vi "LightSheet.vi"() -> ()   [LabVIEW 2015]
uses:
  Camera Properties.ctl
  ModeEnum.ctl
  CameraState.ctl
  Stack_State.ctl
  Stack Track.ctl
  CameraControlTypeDef.ctl
  <vilib>/DAQmx/write.llb/DAQmx Write (Digital 1D Wfm NChan NSamp).vi
  <vilib>/DAQmx/write.llb/DAQmx Write (Analog 1D Wfm NChan NSamp).vi
  <vilib>/DAQmx/create/channels.llb/DAQmx Create Channel (AO-Voltage-Basic).vi
  <vilib>/DAQmx/configure/timing.llb/DAQmx Timing (Sample Clock).vi
  <vilib>/Waveform/DWDTOps.llb/DWDT Uncompress Digital.vi
  <vilib>/DAQmx/miscellaneous.llb/DAQmx Fill In Error Info.vi
  <vilib>/vision/NI_Vision_Development_Module.lvlib
panel:
  in  "Tab Control":enum32{"Camera Settings", "Recording"}(tab)
  in  "Scan":bool
  in  "Scan Continuously":bool
  in  "Camera Mode":T1(ring)
  in  "Slit Width /percent":dbl=100.0
  out "error IO":errorcluster
  in  "V Height":dbl=2048.0 min=4.0 max=2048.0 step=4.0
  in  "V Offset":dbl min=0.0 max=0.0 step=4.0
  in  "H Offset":dbl min=0.0 max=0.0 step=4.0
  in  "H Width":dbl min=4.0 max=2048.0 step=4.0
  in  "Exposure /ms":dbl=40.0 min=0.0010036691729323308 max=10.000004210526315 step=1e-08
  in  "Trigger Source":dbl(ring)=2.0 items=["Internal"=1.0, "External"=2.0]
  in  "Readout Direction":dbl(ring)=2.0 items=["Forward"=1.0, "Backward"=2.0]
  in  "Scanning Mode":dbl(ring)=12.0 items=["Full Frame"=1.0, "Slit Scanning"=12.0]
  in  "Advanced DCAM Controls":i32(listbox) caption="Multicolumn Listbox"
  in  "Mode":T2
  in  "FOV /um":dbl(slide) scale=-10.0..10.0
  in  "Properties":T3=4211904 items=["SENSOR MODE"=4212128, "CCD MODE"=4212384, "READOUT MODE"=4211872, "ACTIVE VIEW INDEX"=4343136, "BITS PER CHANNEL"=4342976, "IMAGE PIXEL TYPE"=4343296, "BINNING"=4215968, "EXPOSURE TIME"=2049184, "CONTRAST GAIN"=3163312, "CONTRAST OFFSET"=3163328, "LIGHT MODE"=2114720, "SENSITIVITY"=2114992, "PHOTON IMAGING MODE"=2115200, "HIGH DYNAMIC RANGE MODE"=3163360, "WHITE BALANCE"=3163568, "TEMPERATURE"=2115232, "TEMPERATURE TARGET"=2115264, "SENSOR COOLER FAN"=2115296, "LINEBUNDLE HEIGHT"=4212192, "MECHANICAL SHUTTER"=2115488, "BACK FOCUS POSITION"=8422304, "TRIGGER CONNECTOR"=1066432, "TRIGGER SOURCE"=1066144, "OUTPUT TRIGGER SOURCE"=1852576, "TRIGGER GLOBAL EXPOSURE"=2049680, "FIRST TRIGGER BEHAVIOR"=2049696, "CHANNEL SYNC"=1852352, "READOUT DIRECTION"=4211904, "PRE HSYNC COUNT"=1852704, "INTERNAL LINE SPEED"=4191408, "INTERNAL LINE INVERVAL"=4191424]
  out "Image":T4(plugin-control)
  out "Histogram":T5(graph)
  in  "stop":bool
  in  "Calibration":bool
  in  "MultiD Scan":bool
  in  "Stage Controller":bool
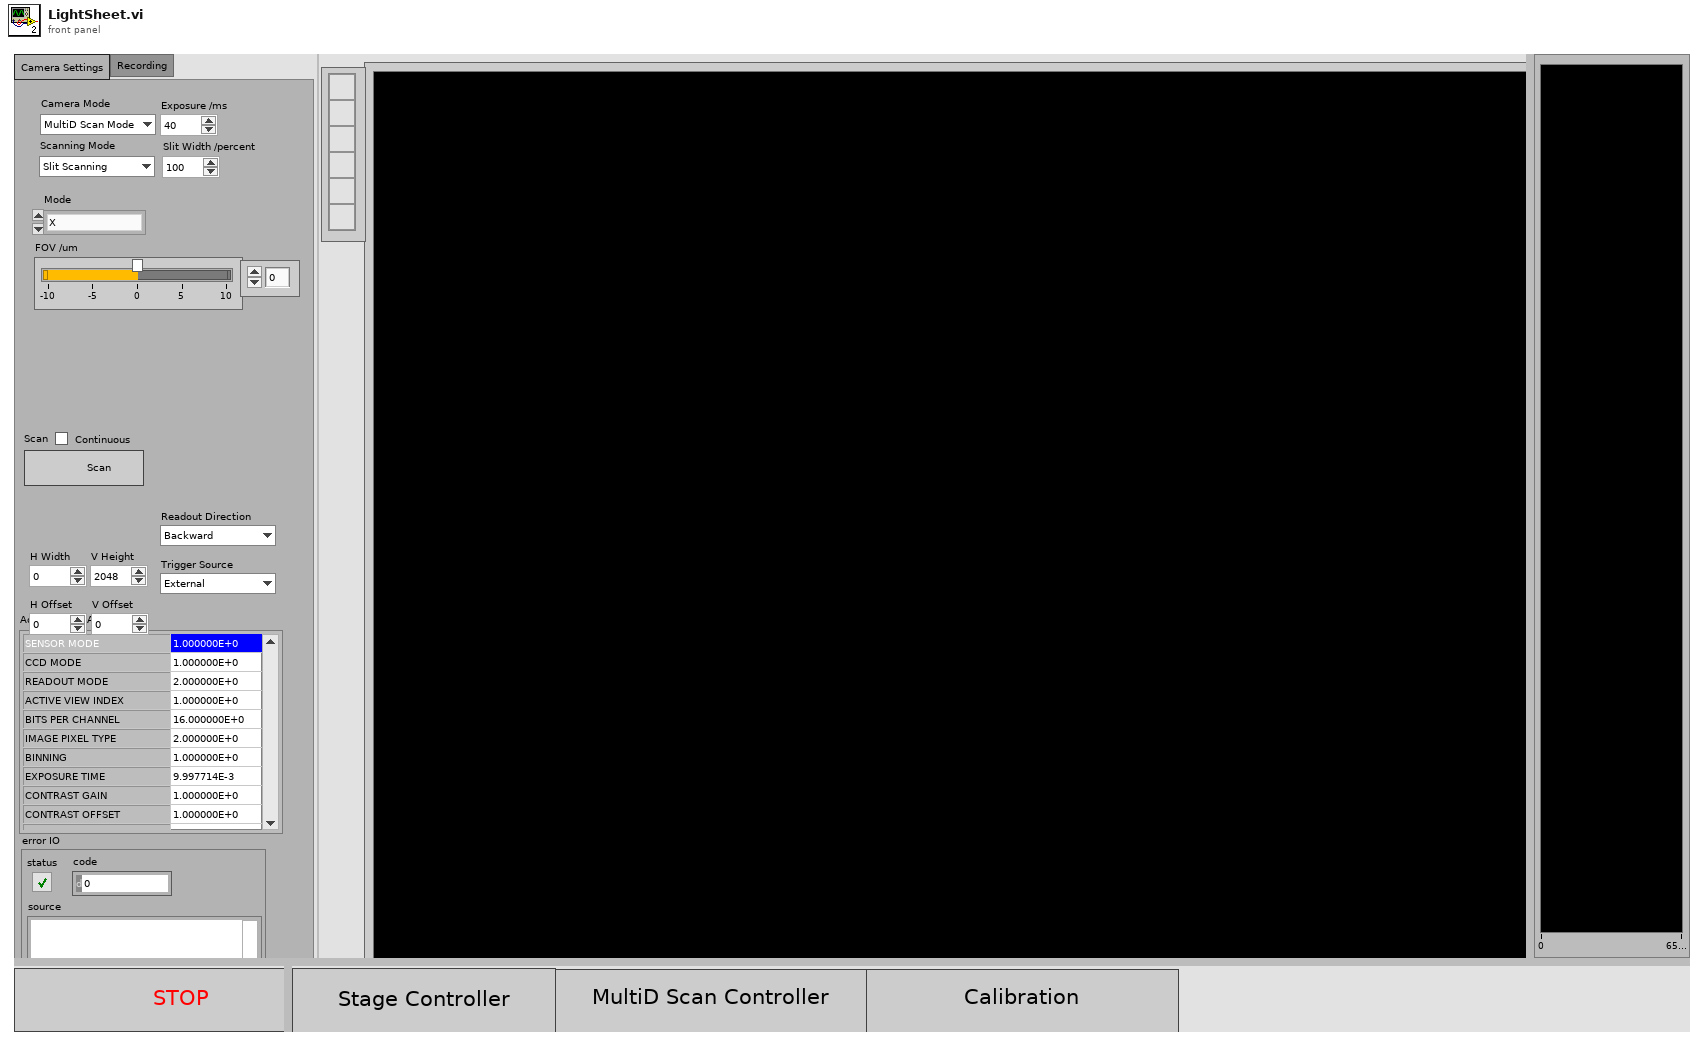
[diagram p1: front panel]
types:
  T1 = enum16{"MultiD Scan Mode", "2D Scan Mode", "Calibration Mode"}
  T2 = typedef "ModeEnum.ctl" = enum16{"X", "XY", "XYZ", "XYZT", "runWaves", "generateWaves", "deInit", "Init", "Idle"}
  T3 = typedef "Camera Properties.ctl" = u32
  T4 = typedef "IMAQ Image.ctl" = refnum<image>
  T5 = cluster{"Starting Value":sgl, "Incremental Value":sgl, "Histogram":u32[]}
  T6 = cluster{"Piezo Position /um":dbl, "Exposure/ms":dbl, "Samples/millisecond":dbl, "Relax/ms":dbl}
  T7 = typedef "CameraControlTypeDef.ctl" = enum16{"IntervalLineInt", "Ram Record", "HardDisk Record", "Disengage Update", "Update", "Idle", "ROI", "Binning", "Scan Mode", "Trigger Mode", "Readout Mode", "Readout Direction", "Preview", "ROIWindow", "Trigger Source"}
  T8 = cluster{"height":u32, "width":u32, "datatype":u32}
  T9 = typedef "Stack_State.ctl" = cluster{"State":T10, "Stack Number":i32, "Image":u16[][], "Stacks":i32}
  T10 = typedef "Stack Track.ctl" = enum16{"Idle", "Display", "Start Sequence", "Read Disk", "STOP", "Collecting", "End"}
  T11 = typedef "CameraState.ctl" = enum16{"init", "active", "deinit"}
  T12 = cluster{"Mode":T2, cluster{"Piezo Position /um":dbl, "Exposure/ms":dbl, "Samples/millisecond":dbl, "Relax/ms":dbl}}
  T13 = typedef "Image Type" = u32
  T14 = cluster{"Value":i32, "Minimum":i32, "Maximum":i32, "Increment":i32}
  T15 = cluster{"Minimum":i32, "Maximum":i32, "Increment":i32}
  T16 = cluster{"Enum":T7, dbl, "timeout in ms (-1)":u32}
  T17 = cluster{"State":T10, "Timeout":i32, "Data 16":u16[][], "Timeout":i32}
  T18 = cluster{"Enum":T7, "Trigger Source":dbl, "timeout in ms (-1)":i32}
  T19 = cluster{"Enum":T7, "Exposure /ms":dbl, "Parameter":u32}
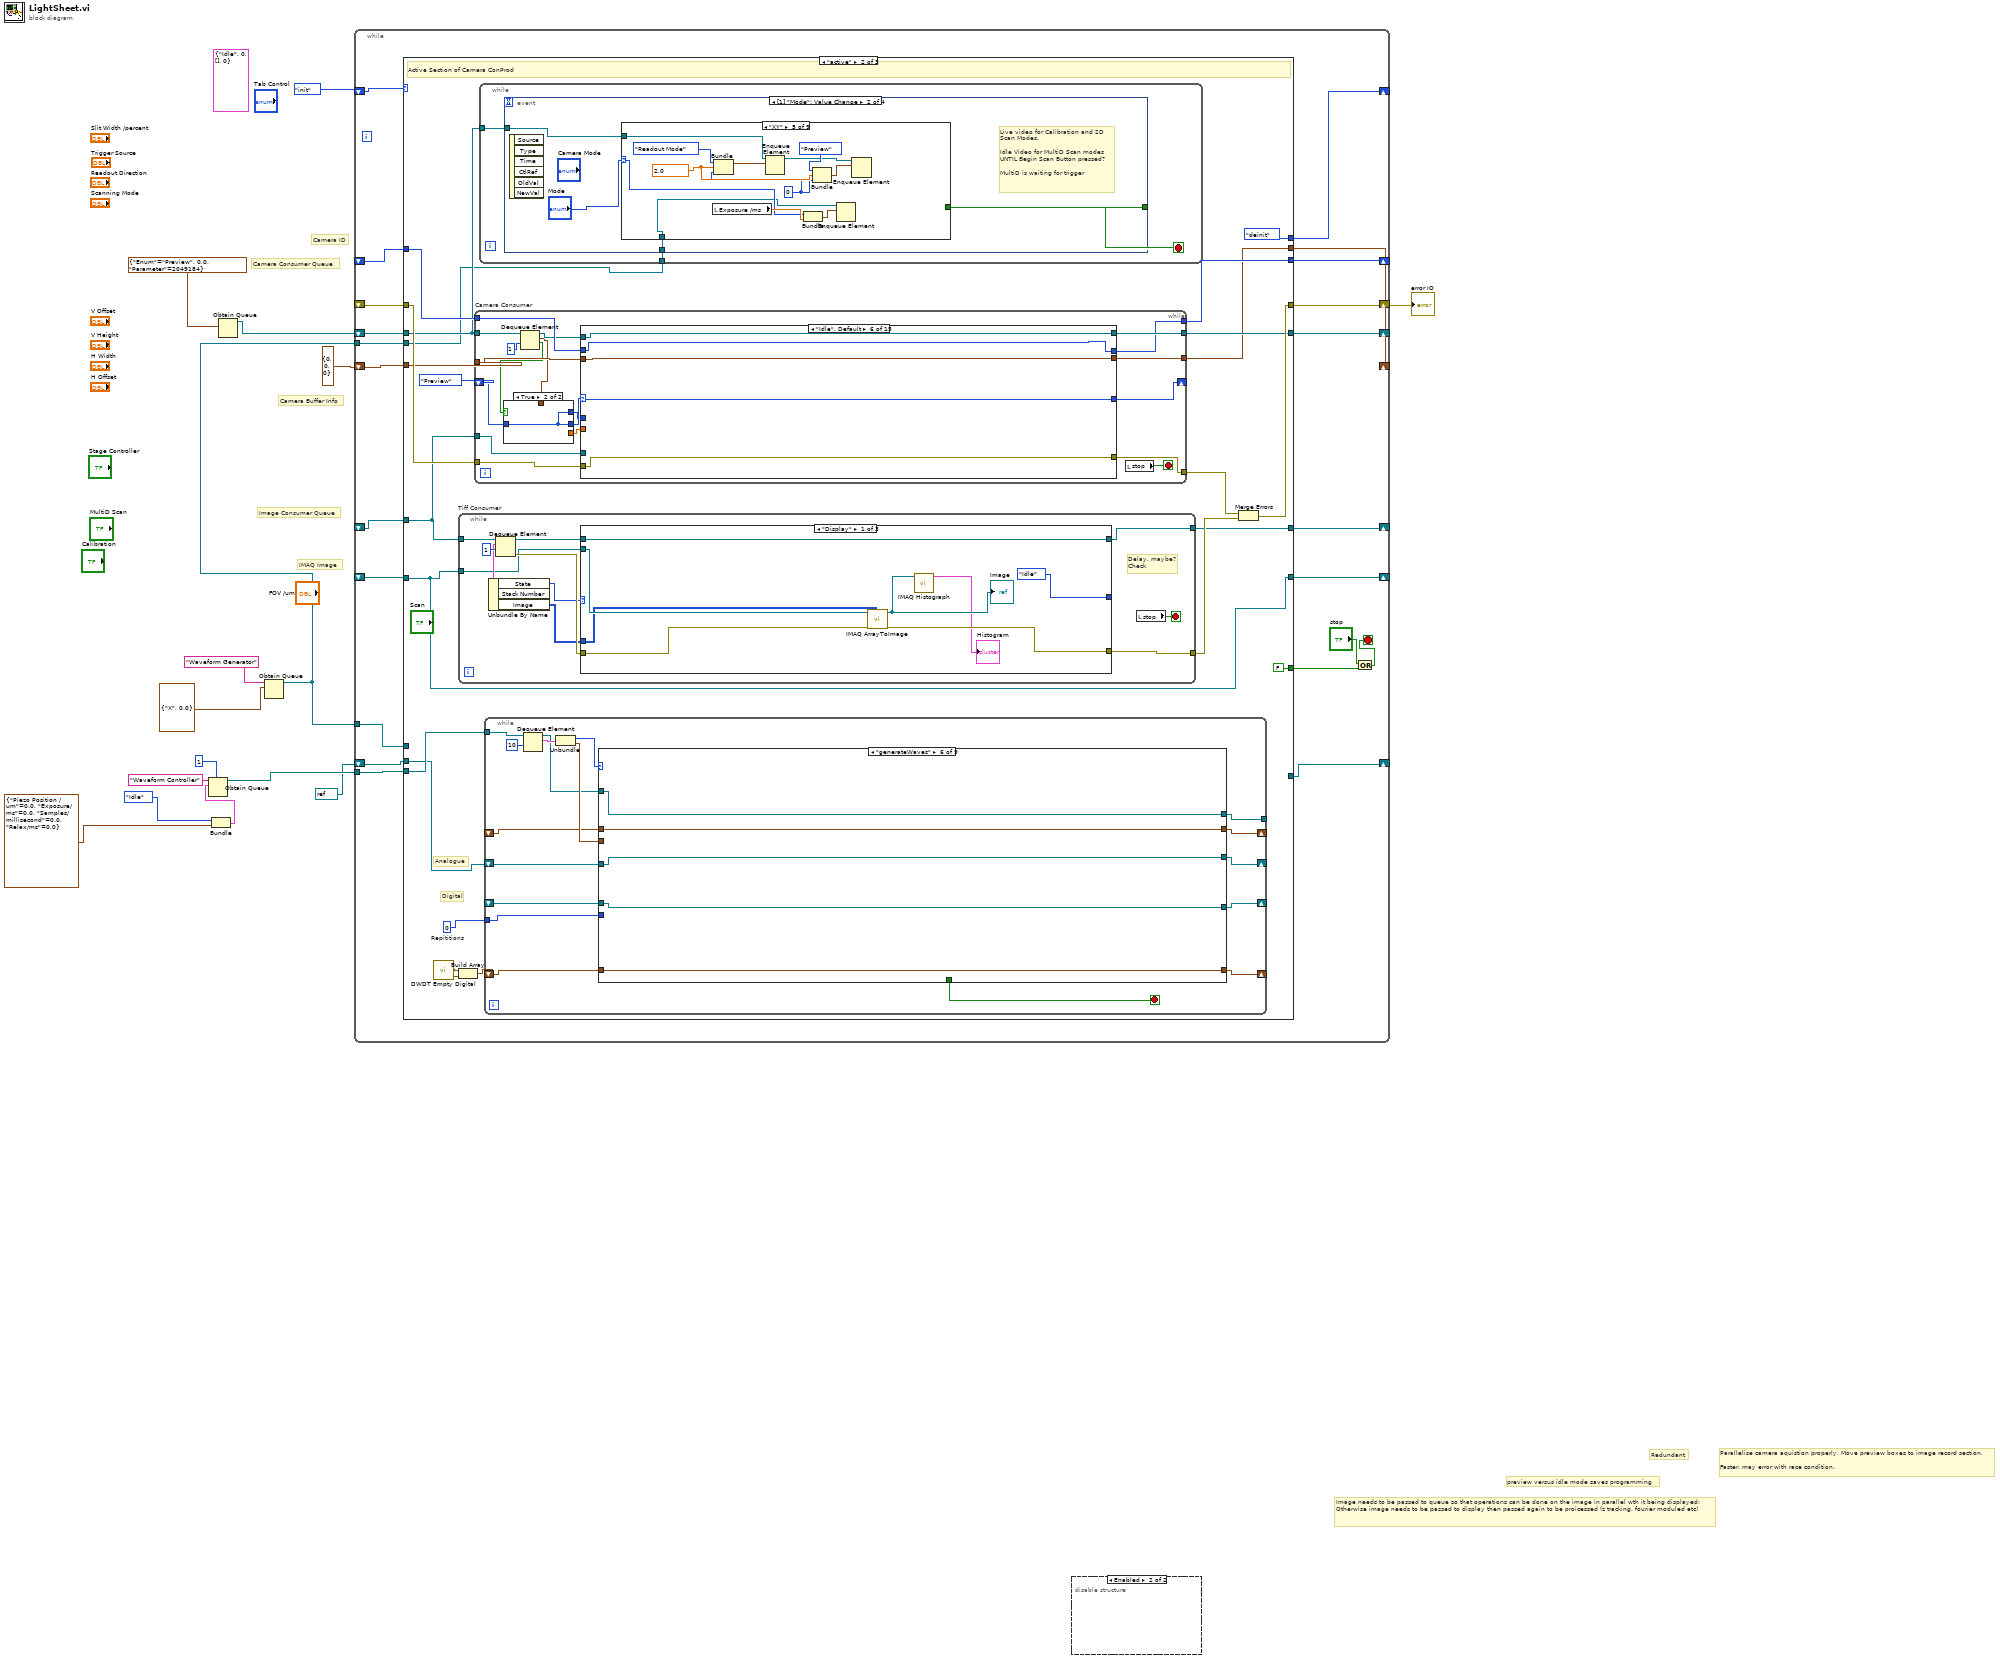
[diagram p0: block diagram]
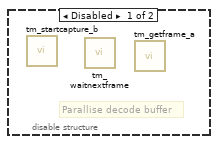
[diagram p2: hidden frame]
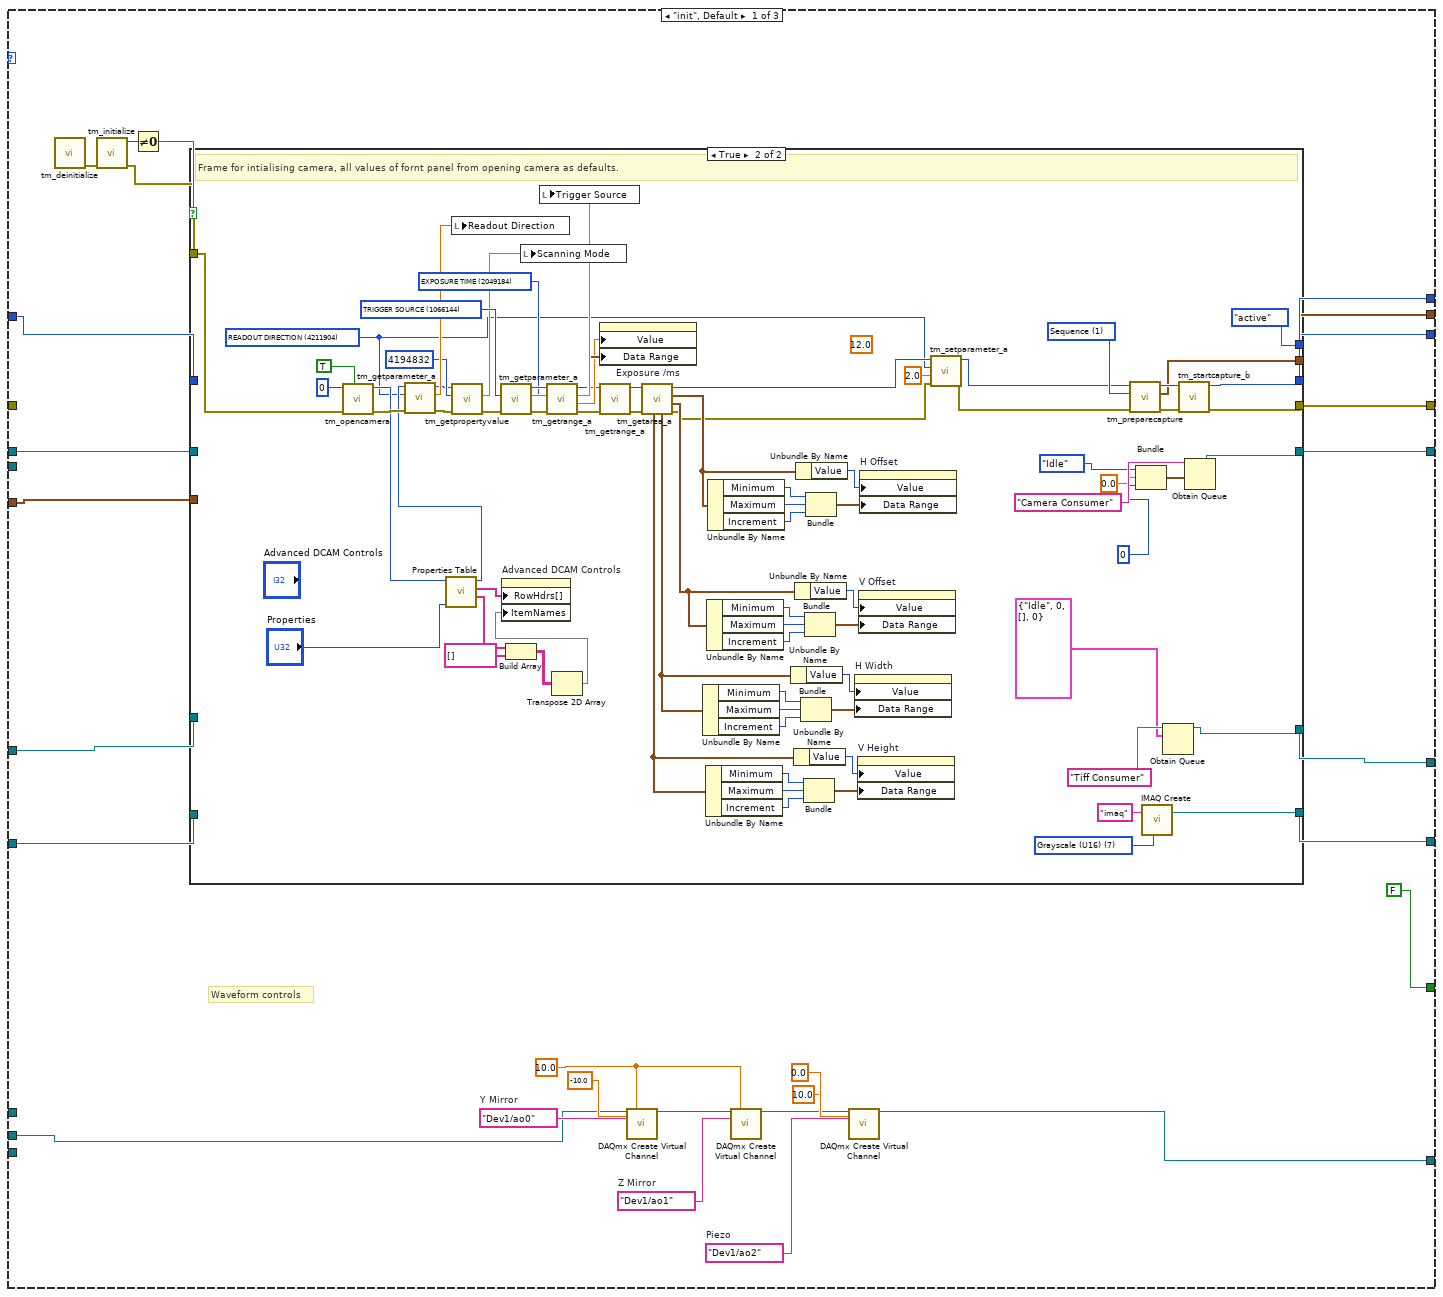
[diagram p3: hidden frame]
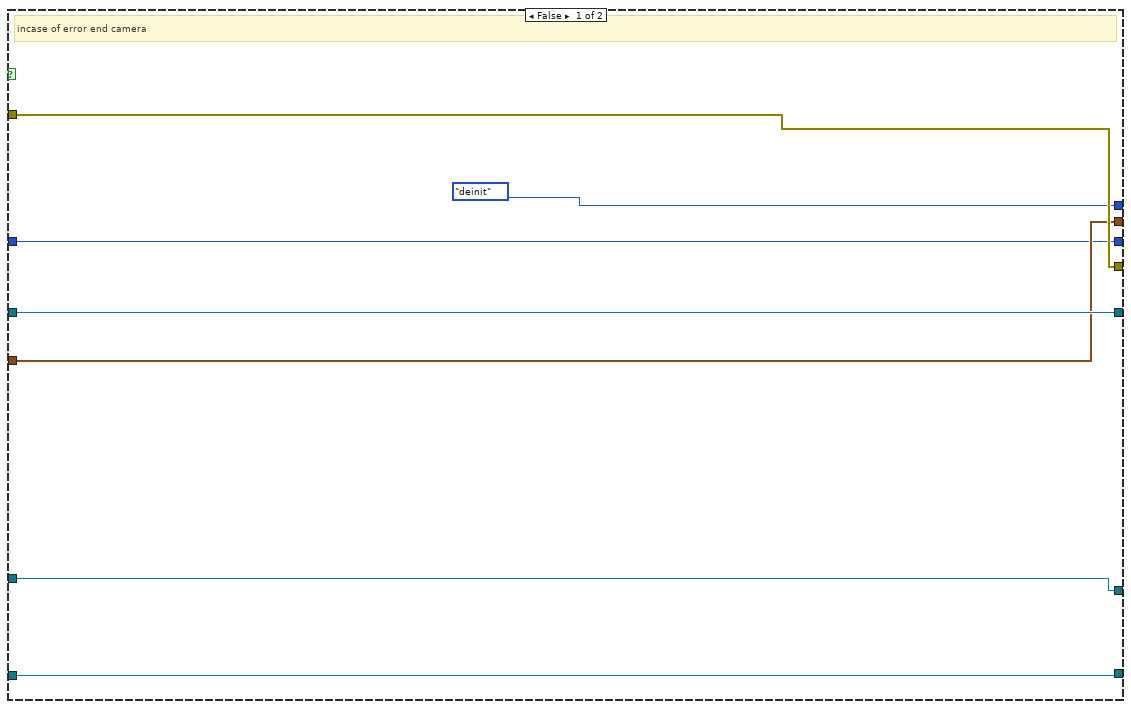
[diagram p4: hidden frame]
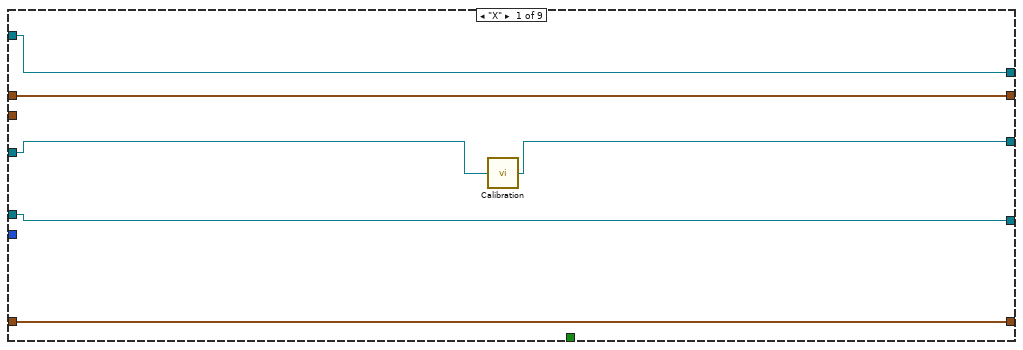
[diagram p5: hidden frame]
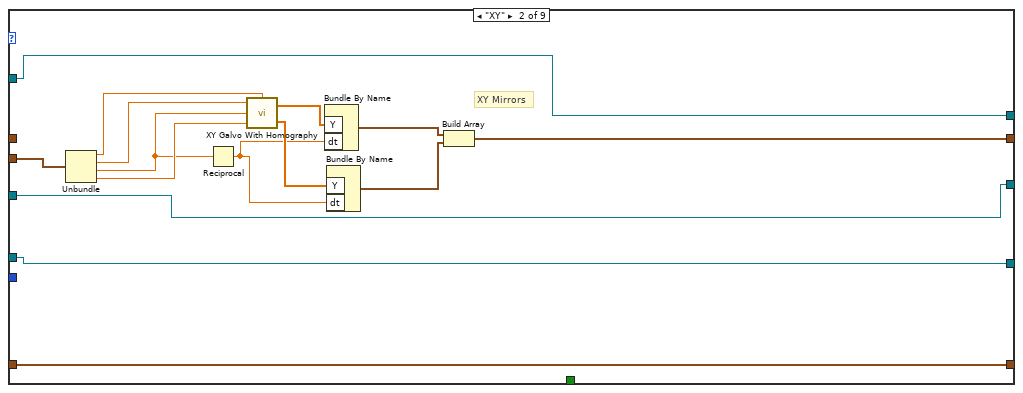
[diagram p6: hidden frame]
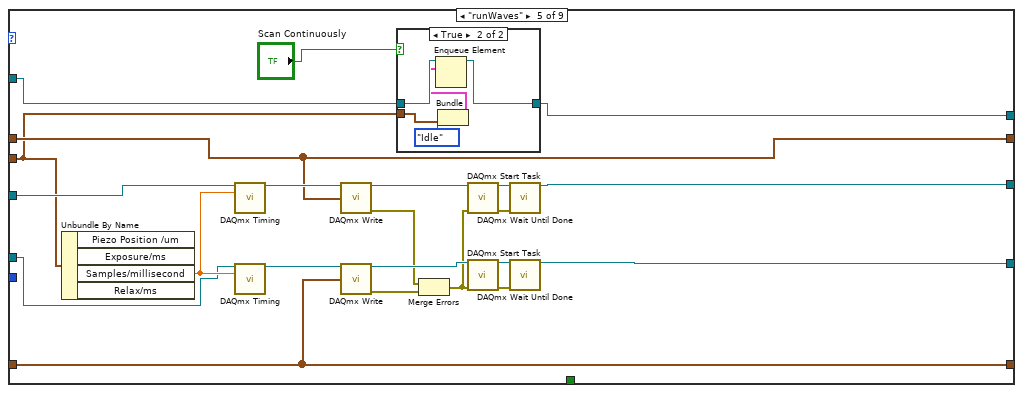
[diagram p9: hidden frame]
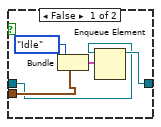
[diagram p10: hidden frame]
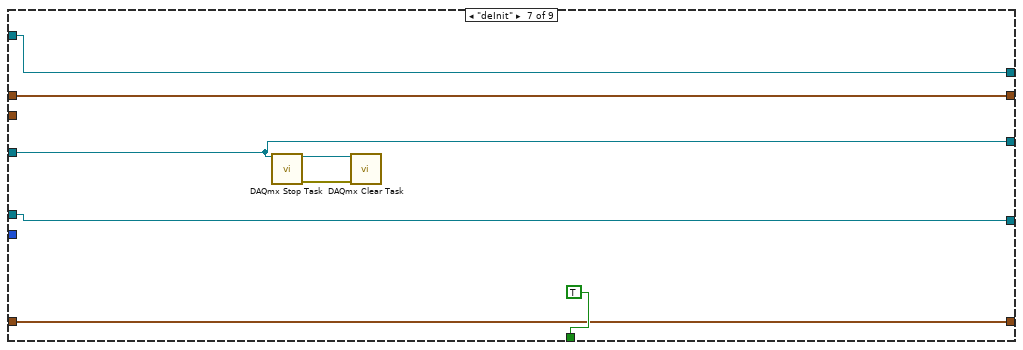
[diagram p11: hidden frame]
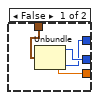
[diagram p16: hidden frame]
diagram:
  (unwired) T9 {"State"=enum."Idle", "Stack Number"=0, "Image"=[], "Stacks"=0} ("input cluster")
  # "IMAQ Image"
  # "Camera Buffer Info"
  # "Image needs to be passed to queue so that operations can be done on the image in parallel wth it being displayed;\nOtherwise image needs to be passed to display then passed again to be proicessed (z tracking, fourier moduled etc)"
  # "preview versus idle mode saves programming"
  # "Parallelise camera aquistion properly. Move preview boxes to image record section.\n\nFaster. may error with race condition."
  # "Redundant"
  # "Image Consumer Queue"
  # "Camera Consumer Queue"
  # "Camera ID"
  n1 = Bundle("Mode"=ModeEnum."Idle", T6 {"Piezo Position /um"=0.0, "Exposure/ms"=0.0, "Samples/millisecond"=0.0, "Relax/ms"=0.0}) -> (w6:T12)  [unwired: 1 in]
  n2 = Obtain Queue(max queue size (-1, unlimited)=1, name (unnamed)="Waveform Controller", element data type=w6) -> (queue out=w3:refnum<queue>)  [unwired: 2 in, 2 out]
  n3 = Obtain Queue(element data type=cluster{"Enum":T7, dbl, "Parameter":u32} {"Enum"=enum."Preview", 0.0, "Parameter"=2049184}) -> (queue out=w10:refnum<queue>)  [unwired: 4 in, 2 out]
  n4 = Obtain Queue(name (unnamed)="Waveform Generator", element data type=cluster{"Mode":T2, "Exposure":dbl} {"Mode"=enum."X", "Exposure"=0.0}) -> (queue out=w9:refnum<queue>)  [unwired: 3 in, 2 out]
  n5 = while {
    shift-right: [w37] -> _
    shift-left: CameraState."init" -> [w36]
    shift-right: [w35] -> _
    shift-left: _ -> [w34]
    shift-right: [w33] -> w14
    shift-left: _ -> [w32]
    shift-right: [w30] -> _
    shift-left: _ -> [w29]
    shift-right: [w31] -> _
    shift-left: w10 -> [w28]
    shift-right: [w24] -> _
    shift-left: T8 {"height"=0, "width"=0, "datatype"=0} ("Buffer Info") -> [w23]
    shift-right: [w22] -> _
    shift-left: _ -> [w21]
    tunnel: w9 -> [w20]
    tunnel: w9 -> [w19]
    tunnel: w3 -> [w18]
    shift-right: [w17] -> _
    shift-left: refnum<k21> refnum ("Mirror Z 2") -> [w16]
    stop <- w26 stop-if-true
    n6 = case shown="\"active\"" w36 {
      tunnel: [w61 CameraState."deinit" CameraState."init"] -> w37
      tunnel: [w60 w171 w475] -> w35
      tunnel: w34 -> [w51 w172 w475]
      tunnel: [w59 w170 w478] -> w33
      tunnel: w32 -> [_ w164 w479]
      tunnel: [w58 w167 w472] -> w31
      tunnel: [w57 w166 w473] -> w30
      tunnel: w29 -> [w55 w159 w473]
      tunnel: w28 -> [w56 w157 w472]
      tunnel: [FALSE ("stop") FALSE ("stop") TRUE ("stop")] -> w25
      tunnel: [w53 w162 w470] -> w24
      tunnel: w23 -> [w52 w161 w470]
      tunnel: w21 -> [w49 w158 w469]
      tunnel: [w50 w158 w469] -> w22
      tunnel: w20 -> [_ _ _]
      tunnel: w19 -> [_ w156 _]
      tunnel: [w41 _ w467] -> w17
      tunnel: w18 -> [_ w152 _]
      tunnel: w16 -> [w38 w151 w467]
      frame "init", Default {
        w44 = tag "Dev1/ao2"  # Piezo
        w45 = tag "Dev1/ao1"  # Z Mirror
        w46 = tag "Dev1/ao0"  # Y Mirror
        w48 = 10.0 ("maximum value")
        # "Waveform controls"
        n7 = call "tm_deinitialize.vi"() -> ("error out"=w65:errorcluster)  [unwired: 11 in]
        n8 = call "tm_initialize.vi"("error in (no error)"=w65) -> ("error out"=w62:errorcluster, "Number Of Cameras"=w64:u32)  [unwired: 7 in, 2 out]
        n9 = Not Equal To 0?(x=w64) -> (x != 0?=w63:bool)
        n10 = case shown="True" w63 {
          tunnel: w62 -> [w72 w144]
          tunnel: [CameraState."deinit" CameraState."active"] -> w61
          tunnel: [w72 w127] -> w59
          tunnel: [w67 w125] -> w60
          tunnel: [w70 w99] -> w58
          tunnel: [w69 w97] -> w57
          tunnel: w56 -> [w70 _]
          tunnel: w55 -> [w69 _]
          tunnel: [w68 w87] -> w53
          tunnel: w52 -> [w68 _]
          tunnel: w51 -> [w67 _]
          tunnel: [w66 w84] -> w50
          tunnel: w49 -> [w66 _]
          frame False {
            # "incase of error end camera"
          }
          frame True {
            (unwired) 12.0 ("Value in")
            w86 = T13 7 items=["Grayscale (U8)", "Grayscale (I16)", "Grayscale (SGL)", "Complex (CSG)", "RGB (U32)", "HSL (U32)", "RGB (U64)", "Grayscale (U16)"] ("Image Type")
            w129 = 1 items=["Snap", "Sequence"] ("Capture mode")
            w141 = u32 2049184 items=["SENSOR MODE"=4212128, "CCD MODE"=4212384, "READOUT MODE"=4211872, "ACTIVE VIEW INDEX"=4343136, "BITS PER CHANNEL"=4342976, "IMAGE PIXEL TYPE"=4343296, "BINNING"=4215968, "EXPOSURE TIME"=2049184, "CONTRAST GAIN"=3163312, "CONTRAST OFFSET"=3163328, "LIGHT MODE"=2114720, "SENSITIVITY"=2114992, "PHOTON IMAGING MODE"=2115200, "HIGH DYNAMIC RANGE MODE"=3163360, "WHITE BALANCE"=3163568, "TEMPERATURE"=2115232, "TEMPERATURE TARGET"=2115264, "SENSOR COOLER FAN"=2115296, "LINEBUNDLE HEIGHT"=4212192, "MECHANICAL SHUTTER"=2115488, "BACK FOCUS POSITION"=8422304, "TRIGGER CONNECTOR"=1066432, "TRIGGER SOURCE"=1066144, "OUTPUT TRIGGER SOURCE"=1852576, "TRIGGER GLOBAL EXPOSURE"=2049680, "FIRST TRIGGER BEHAVIOR"=2049696, "CHANNEL SYNC"=1852352, "READOUT DIRECTION"=4211904, "PRE HSYNC COUNT"=1852704, "INTERNAL LINE SPEED"=4191408, "INTERNAL LINE INVERVAL"=4191424] ("Parameter")
            w79 = T3 4211904 items=["SENSOR MODE"=4212128, "CCD MODE"=4212384, "READOUT MODE"=4211872, "ACTIVE VIEW INDEX"=4343136, "BITS PER CHANNEL"=4342976, "IMAGE PIXEL TYPE"=4343296, "BINNING"=4215968, "EXPOSURE TIME"=2049184, "CONTRAST GAIN"=3163312, "CONTRAST OFFSET"=3163328, "LIGHT MODE"=2114720, "SENSITIVITY"=2114992, "PHOTON IMAGING MODE"=2115200, "HIGH DYNAMIC RANGE MODE"=3163360, "WHITE BALANCE"=3163568, "TEMPERATURE"=2115232, "TEMPERATURE TARGET"=2115264, "SENSOR COOLER FAN"=2115296, "LINEBUNDLE HEIGHT"=4212192, "MECHANICAL SHUTTER"=2115488, "BACK FOCUS POSITION"=8422304, "TRIGGER CONNECTOR"=1066432, "TRIGGER SOURCE"=1066144, "OUTPUT TRIGGER SOURCE"=1852576, "TRIGGER GLOBAL EXPOSURE"=2049680, "FIRST TRIGGER BEHAVIOR"=2049696, "CHANNEL SYNC"=1852352, "READOUT DIRECTION"=4211904, "PRE HSYNC COUNT"=1852704, "INTERNAL LINE SPEED"=4191408, "INTERNAL LINE INVERVAL"=4191424] ("Parameter")
            w147 = u32 1066144 items=["SENSOR MODE"=4212128, "CCD MODE"=4212384, "READOUT MODE"=4211872, "ACTIVE VIEW INDEX"=4343136, "BITS PER CHANNEL"=4342976, "IMAGE PIXEL TYPE"=4343296, "BINNING"=4215968, "EXPOSURE TIME"=2049184, "CONTRAST GAIN"=3163312, "CONTRAST OFFSET"=3163328, "LIGHT MODE"=2114720, "SENSITIVITY"=2114992, "PHOTON IMAGING MODE"=2115200, "HIGH DYNAMIC RANGE MODE"=3163360, "WHITE BALANCE"=3163568, "TEMPERATURE"=2115232, "TEMPERATURE TARGET"=2115264, "SENSOR COOLER FAN"=2115296, "LINEBUNDLE HEIGHT"=4212192, "MECHANICAL SHUTTER"=2115488, "BACK FOCUS POSITION"=8422304, "TRIGGER CONNECTOR"=1066432, "TRIGGER SOURCE"=1066144, "OUTPUT TRIGGER SOURCE"=1852576, "TRIGGER GLOBAL EXPOSURE"=2049680, "FIRST TRIGGER BEHAVIOR"=2049696, "CHANNEL SYNC"=1852352, "READOUT DIRECTION"=4211904, "PRE HSYNC COUNT"=1852704, "INTERNAL LINE SPEED"=4191408, "INTERNAL LINE INVERVAL"=4191424] ("Parameter")
            # "Frame for intialising camera, all values of fornt panel from opening camera as defaults."
            n11 = call "tm_opencamera.vi"("Force Open"=TRUE, "error in (no error)"=w144, "Camera Index"=u32 0) -> ("error out"=w148:errorcluster, "Handle out"=w95:u32)  [unwired: 6 in, 1 out]
            n12 = call "Properties Table.vi"("Properties"="Properties", "Handle In"=w95) -> ("Value Stirngs Out"=w92:string[], "Row Headers"=w93:string[], "Handle Out"=w94:u32)  [unwired: 3 in, 1 out]
            n13 = call "tm_getparameter_a.vi"("error in (no error)"=w148, "Parameter"=w79, "Handle in"=w94) -> ("error out"=w130:errorcluster, "Value out"=w145:dbl, "Handle out"=w133:u32)  [unwired: 6 in]
            n14 = local write "Readout Direction"(w145) -> ()
            n15 = call "tm_getpropertyvalue.vi"("error in (no error)"=w130, "Property ID"=u32 4194832, "Handle in"=w133) -> ("error out"=w131:errorcluster, "Value in"=w132:sgl)  [unwired: 6 in, 1 out]
            n16 = call "tm_getparameter_a.vi"("error in (no error)"=w131, "Parameter"=w147) -> ("error out"=w142:errorcluster, "Value out"=w146:dbl, "Handle out"=w143:u32)  [unwired: 7 in]
            n17 = Build Array(w92, string[] [] ("element")) -> (w90:string[][])
            n18 = local write "Scanning Mode"(w132) -> ()
            n19 = local write "Trigger Source"(w146) -> ()
            n20 = call "tm_getrange_a.vi"("error in (no error)"=w142, "Parameter"=w141, "Handle in"=w143) -> ("error out"=w137:errorcluster, "default"=w139:dbl, "Range"=w140:cluster{"min":dbl, "max":dbl, "step":dbl}, "Handle out"=w138:u32)  [unwired: 2 in, 3 out]
            n21 = Transpose 2D Array(2D array=w90) -> (transposed array=w89:string[][])
            n22 = property on="Advanced DCAM Controls" class="MCListbox (strict)"("RowHdrs[]"=w93, "ItemNames"=w89) -> ()  [unwired: 2 in, 2 out]
            n23 = property on="Exposure /ms" class="DigNum (strict)"("Value"=w139, "Data Range"=w140) -> ()  [unwired: 2 in, 2 out]
            n24 = call "tm_getrange_a.vi"("error in (no error)"=w137, "Handle in"=w138) -> ("error out"=w136:errorcluster, "Handle out"=w135:u32)  [unwired: 3 in, 5 out]
            n25 = call "tm_getarea_a.vi"("error in (no error)"=w136, "Handle in"=w135) -> ("error out"=w81:errorcluster, "V Offset"=w101:T14, "H Offset"=w124:T14, "Handle out"=w83:u32, "H Width"=w102:T14, "V Width"=w103:T14)  [unwired: 4 in]
            n26 = Unbundle By Name(w102) -> ("Minimum"=w113:i32, "Maximum"=w112:i32, "Increment"=w111:i32)
            n27 = Unbundle By Name(w103) -> ("Minimum"=w104:i32, "Maximum"=w105:i32, "Increment"=w106:i32)
            n28 = Unbundle By Name(w101) -> ("Minimum"=w114:i32, "Maximum"=w115:i32, "Increment"=w116:i32)
            n29 = Unbundle By Name(w124) -> ("Minimum"=w123:i32, "Maximum"=w122:i32, "Increment"=w121:i32)
            n30 = Unbundle By Name(w102) -> ("Value"=w109:i32)
            n31 = Unbundle By Name(w103) -> ("Value"=w108:i32)
            n32 = Unbundle By Name(w101) -> ("Value"=w118:i32)
            n33 = Unbundle By Name(w124) -> ("Value"=w119:i32)
            n34 = Bundle("Minimum"=w113, "Maximum"=w112, "Increment"=w111) -> (w110:T15)  [unwired: 1 in]
            n35 = Bundle("Minimum"=w104, "Maximum"=w105, "Increment"=w106) -> (w107:T15)  [unwired: 1 in]
            n36 = Bundle("Minimum"=w114, "Maximum"=w115, "Increment"=w116) -> (w117:T15)  [unwired: 1 in]
            n37 = Bundle("Minimum"=w123, "Maximum"=w122, "Increment"=w121) -> (w120:T15)  [unwired: 1 in]
            n38 = property on="H Width" class="DigNum (strict)"("Value"=w109, "Data Range"=w110) -> ()  [unwired: 2 in, 2 out]
            n39 = property on="V Height" class="DigNum (strict)"("Value"=w108, "Data Range"=w107) -> ()  [unwired: 2 in, 2 out]
            n40 = property on="V Offset" class="DigNum (strict)"("Value"=w118, "Data Range"=w117) -> ()  [unwired: 2 in, 2 out]
            n41 = property on="H Offset" class="DigNum (strict)"("Value"=w119, "Data Range"=w120) -> ()  [unwired: 2 in, 2 out]
            n42 = call "tm_setparameter_a.vi"("error in (no error)"=w81, "Value in"=2.0, "Parameter"=w79, "Handle in"=w83) -> ("error out"=w80:errorcluster, "Handle out"=w82:u32)  [unwired: 6 in]
            n43 = call "tm_preparecapture.vi"("error in (no error)"=w80, "Capture mode"=w129, "Handle in"=w82) -> ("error out"=w128:errorcluster, "Buffer Info"=w87:T8, "Handle out"=w126:u32)  [unwired: 5 in, 1 out]
            n44 = Bundle("Enum"=CameraControlTypeDef."Idle", 0.0, "timeout in ms (-1)"=u32 0) -> (w75:T16)  [unwired: 1 in]
            n45 = call "IMAQ Create"("Image Name"="imaq", "Image Type"=w86) -> ("New Image"=w84:T4)  [unwired: 3 in, 1 out]
            n46 = Obtain Queue(name (unnamed)="Tiff Consumer", element data type=T9 {"State"=enum."Idle", "Stack Number"=0, "Image"=[], "Stacks"=0} ("input cluster")) -> (queue out=w97:refnum<queue>)  [unwired: 3 in, 2 out]
            n47 = call "tm_startcapture_b.vi"("error in (no error)"=w128, "Handle in"=w126) -> ("error out"=w127:errorcluster, "Handle out"=w125:u32)  [unwired: 8 in]
            n48 = Obtain Queue(name (unnamed)="Camera Consumer", element data type=w75) -> (queue out=w99:refnum<queue>)  [unwired: 3 in, 2 out]
          }
        }
        n49 = call-poly <vilib>:"DAQmx Create Virtual Channel.vi"("task in"=w38, "maximum value"=w48, "minimum value"=-10.0, "physical channels"=w46) -> ("task out"=w40:refnum<k21>)  [unwired: 10 in, 1 out]
        n50 = call-poly <vilib>:"DAQmx Create Virtual Channel.vi"("task in"=w40, "maximum value"=w48, "physical channels"=w45) -> ("task out"=w39:refnum<k21>)  [unwired: 11 in, 1 out]
        n51 = call-poly <vilib>:"DAQmx Create Virtual Channel.vi"("task in"=w39, "maximum value"=10.0 ("minimum value"), "minimum value"=0.0 ("maximum value"), "physical channels"=w44) -> ("task out"=w41:refnum<k21>)  [unwired: 10 in, 1 out]
      }
      frame "active" {
        w155 = 0  # Repititions
        # "Digital"
        # "Analogue"
        # "Active Section of Camera ConProd"
        n52 = call <vilib>:"DWDT Empty Digital.vi"() -> ("digital waveform out"=w153:digitalwaveform)  [unwired: 5 in]
        n53 = while "Tiff Consumer" {
          tunnel: [w279] -> w169
          tunnel: [w282] -> w166
          tunnel: w159 -> [w284]
          tunnel: w158 -> [w276]
          stop <- w286 stop-if-true
          # "Delay, maybe?\nCheck"
          n54 = Dequeue Element(queue=w284, timeout in ms (-1)=1) -> (queue out=w281:refnum<queue>, element=w283:T9, error out=w280:errorcluster)  [unwired: 1 in, 1 out]
          n55 = Unbundle By Name(w283) -> ("State"=w277:T10, "Image"=w278:u16[][])  [unwired: 1 out]
          n56 = case shown="\"Display\"" w277 {
            selector: w277 -> [_ w297 w298]
            tunnel: [w294 w296 w299] -> w282
            tunnel: w281 -> [w294 w296 w299]
            tunnel: [Stack_Track."Idle" ("State") w297 w298] -> _
            tunnel: w278 -> [w289 _ _]
            tunnel: w276 -> [w293 _ _]
            tunnel: w280 -> [w292 w295 w300]
            tunnel: [w291 w295 w300] -> w279
            frame "Display" {
              n57 = call "IMAQ ArrayToImage"("Image Pixels (U16)"=w289, "error in (no error)"=w292, "Image"=w293) -> ("error out"=w291:errorcluster, "Image Out"=w288:T4)  [unwired: 7 in]
              "Image" <- w288
              n58 = call "IMAQ Histograph"("Image"=w288) -> ("Histogram Graph"=→"Histogram":T5)  [unwired: 7 in, 3 out]
            }
            frame "Idle", Default {
            }
            frame "Start Sequence" {
            }
          }
          n59 = local read "stop"() -> (w286:bool)
        }
        n60 = Build Array(w153, w153) -> (w154:digitalwaveform[])
        n61 = while "Camera Consumer" {
          tunnel: w164 -> [w317]
          tunnel: w172 -> [w314]
          tunnel: [w313] -> w171
          tunnel: [w316] -> w168
          tunnel: w157 -> [w309]
          tunnel: [w318] -> w167
          shift-right: [w315] -> _
          shift-left: CameraControlTypeDef."Preview" ("Enum") -> [w305]
          tunnel: [w312] -> w162
          tunnel: w161 -> [w311]
          tunnel: w159 -> [w304]
          stop <- w319 stop-if-true
          n62 = Dequeue Element(queue=w309, timeout in ms (-1)=1) -> (queue out=w308:refnum<queue>, element=w303:cluster{"Enum":T7, dbl, "Parameter":u32}, timed out?=w307:bool)  [unwired: 1 in, 1 out]
          n63 = case shown="True" w307 {
            tunnel: [w322 w324] -> w306
            tunnel: w305 -> [_ w324]
            tunnel: w303 -> [w323 _]
            tunnel: [w321 _] -> w302
            tunnel: [w320 w324] -> w301
            frame False {
              n64 = Unbundle(w323) -> ("Enum"=w322:T7, w321:dbl, "Parameter"=w320:u32)
            }
            frame True {
            }
          }
          n65 = case shown="\"Idle\", Default" w306 {
            selector: w306 -> [w328 w333 w338 w343 w351 w356 w361 w366 w371 w376 w381 w386 _ w405 _]
            tunnel: w308 -> [w327 w334 w339 w344 w352 w357 w362 w367 w372 w377 w382 w387 w402 w407 w412]
            tunnel: [w327 w334 w339 w344 w352 w357 w362 w367 w372 w377 w382 w387 w402 w407 w412] -> w318
            tunnel: w317 -> [w329 w332 w337 w342 w350 w355 w360 w365 w370 w375 w380 w385 w392 w404 w410]
            tunnel: [w329 w332 w337 w342 w350 w355 w360 w365 w370 w375 w380 w385 w396 w404 w410] -> w316
            tunnel: [w328 w333 w338 w343 w351 w356 w361 w366 w371 w376 w381 w386 CameraControlTypeDef."Preview" ("Enum") w405 CameraControlTypeDef."Preview" ("Enum")] -> w315
            tunnel: w314 -> [w326 w331 w336 w341 w348 w354 w359 w364 w369 w374 w379 w384 w400 w406 w411]
            tunnel: [w326 w331 w336 w341 w347 w354 w359 w364 w369 w374 w379 w384 w398 w406 w411] -> w313
            tunnel: [w325 w330 w335 w340 w349 w353 w358 w363 w368 w373 w378 w383 w394 w403 w409] -> w312
            tunnel: w311 -> [w325 w330 w335 w340 w349 w353 w358 w363 w368 w373 w378 w383 w394 w403 w409]
            tunnel: w304 -> [_ _ _ _ _ _ _ _ _ _ _ _ w393 _ _]
            tunnel: w302 -> [_ _ _ _ w345 _ _ _ _ _ _ _ _ _ _]
            tunnel: w301 -> [_ _ _ _ w346 _ _ _ _ _ _ _ _ _ _]
            frame "IntervalLineInt" {
            }
            frame "Ram Record" {
            }
            frame "HardDisk Record" {
            }
            frame "Disengage Update" {
            }
            frame "Update" {
              n66 = call "tm_setparameter_a.vi"("Value in"=w345, "Parameter"=w346, "Handle in"=w348) -> ("Handle out"=w347:u32)  [unwired: 7 in, 1 out]
            }
            frame "Idle", Default {
            }
            frame "ROI" {
            }
            frame "Binning" {
            }
            frame "Scan Mode" {
            }
            frame "Trigger Mode" {
            }
            frame "Readout Mode" {
            }
            frame "Readout Direction" {
            }
            frame "Preview" {
              w389 = 0 ("Timeout")
              n67 = call "tm_waitnextframe.vi"("error in (no error)"=w392, "Timeout"=3000, "Handle in"=w400) -> ("error out"=w397:errorcluster, "Handle out"=w399:u32)  [unwired: 5 in, 2 out]
              n68 = call "tm_getframe_a.vi"("error in (no error)"=w397, "Buffer Info"=w394, "Handle in"=w399) -> ("error out"=w396:errorcluster, "Data 16"=w390:u16[][], "Handle out"=w398:u32)  [unwired: 4 in, 2 out]
              n69 = Bundle("State"=Stack_Track."Display", "Timeout"=w389, "Data 16"=w390, "Timeout"=w389) -> (w388:T17)  [unwired: 1 in]
              n70 = Enqueue Element(queue=w393, element=w388, error in (no error)=w392) -> ()  [unwired: 1 in, 3 out]
            }
            frame "ROIWindow" {
            }
            frame "Trigger Source" {
              n71 = call "tm_unpreparecapture.vi"() -> ()  [unwired: 10 in, 2 out]
              n72 = call "tm_setparameter_a.vi"() -> ()  [unwired: 10 in, 2 out]
              n73 = call "tm_preparecapture.vi"() -> ()  [unwired: 8 in, 4 out]
            }
          }
          n74 = local read "stop"() -> (w319:bool)
        }
        n75 = while {
          tunnel: w157 -> [w414]
          tunnel: w156 -> [w413]
          stop <- w415 stop-if-true
          n76 = event shown="[1] \"Mode\": Value Change" {
            selector: _ -> [_ _ _ _]
            dyn-events: _ -> [_ _ _ _]
            timeout: _ -> [_ _ _ _]
            tunnel: [w416 w417 _ _] -> w415
            tunnel: w414 -> [_ w420 _ w465]
            tunnel: w413 -> [_ w418 _ w462]
            event "stop": Value Change {
              n77 = event-data() -> ()  [unwired: 1 in, 6 out]
              n78 = local read "stop"() -> (w416:bool)
            }
            event Value Change {
              # "Live video for Calibration and 2D\nScan Modes.\n\nIdle Video for MultiD Scan modes\nUNTIL Begin Scan Button pressed?\n\nMultiD is waiting for trigger"
              n79 = event-data() -> ()  [unwired: 1 in, 6 out]
              n80 = case shown="\"XY\"" "Mode" {
                selector: "Mode" -> [w423 _ _ _ w446 _ _ _ _]
                tunnel: w420 -> [w431 w439 _ _ w455 _ _ _ _]
                tunnel: w418 -> [w424 _ w442 _ w445 _ _ _ _]
                tunnel: [_ _ _ _ _ TRUE FALSE _ _] -> w417
                frame "X" {
                  w425 = 0 ("timeout in ms (-1)")
                  w426 = 1.0 items=["Internal"=1.0, "External"=2.0] ("Trigger Source")
                  n81 = Bundle("Enum"=CameraControlTypeDef."Readout Mode", "Trigger Source"=w426, "timeout in ms (-1)"=w425) -> (w430:T18)  [unwired: 1 in]
                  n82 = Enqueue Element(queue=w431, element=w430) -> (queue out=w428:refnum<queue>)  [unwired: 2 in, 2 out]
                  n83 = Bundle("Enum"=CameraControlTypeDef."Preview", "Trigger Source"=w426, "timeout in ms (-1)"=w425) -> (w429:T18)  [unwired: 1 in]
                  n84 = Bundle("Mode"=w423, "Exposure /ms"=0.0) -> (w422:cluster{"Mode":T2, "Exposure /ms":dbl})  [unwired: 1 in]
                  n85 = Enqueue Element(queue=w428, element=w429) -> ()  [unwired: 2 in, 3 out]
                  n86 = Enqueue Element(queue=w424, element=w422) -> ()  [unwired: 2 in, 3 out]
                }
                frame "XYZ" {
                  w433 = 0 ("timeout in ms (-1)")
                  w434 = 2.0 items=["Internal"=1.0, "External"=2.0] ("Trigger Source")
                  n87 = Bundle("Enum"=CameraControlTypeDef."Readout Mode", "Trigger Source"=w434, "timeout in ms (-1)"=w433) -> (w438:T18)  [unwired: 1 in]
                  n88 = Enqueue Element(queue=w439, element=w438) -> (queue out=w437:refnum<queue>)  [unwired: 2 in, 2 out]
                  n89 = Bundle("Enum"=CameraControlTypeDef."Idle", "Trigger Source"=w434, "timeout in ms (-1)"=w433) -> (w436:T18)  [unwired: 1 in]
                  n90 = Enqueue Element(queue=w437, element=w436) -> ()  [unwired: 2 in, 3 out]
                }
                frame "generateWaves" {
                  w444 = ModeEnum."generateWaves"  # Mode
                  n91 = local read "Exposure /ms"() -> (w443:dbl)
                  n92 = Bundle("Mode"=w444, "Exposure /ms"=w443) -> (w441:cluster{"Mode":T2, "Exposure /ms":dbl})  [unwired: 1 in]
                  n93 = Enqueue Element(queue=w442, element=w441) -> ()  [unwired: 2 in, 3 out]
                }
                frame "XYZT" {
                }
                frame "XY" {
                  w449 = 0 ("timeout in ms (-1)")
                  w450 = 2.0 items=["Internal"=1.0, "External"=2.0] ("Trigger Source")
                  n94 = local read "Exposure /ms"() -> (w447:dbl)
                  n95 = Bundle("Enum"=CameraControlTypeDef."Readout Mode", "Trigger Source"=w450, "timeout in ms (-1)"=w449) -> (w454:T18)  [unwired: 1 in]
                  n96 = Enqueue Element(queue=w455, element=w454) -> (queue out=w451:refnum<queue>)  [unwired: 2 in, 2 out]
                  n97 = Bundle("Mode"=w446, "Exposure /ms"=w447) -> (w448:cluster{"Mode":T2, "Exposure /ms":dbl})  [unwired: 1 in]
                  n98 = Bundle("Enum"=CameraControlTypeDef."Preview", "Trigger Source"=w450, "timeout in ms (-1)"=w449) -> (w453:T18)  [unwired: 1 in]
                  n99 = Enqueue Element(queue=w445, element=w448) -> ()  [unwired: 2 in, 3 out]
                  n100 = Enqueue Element(queue=w451, element=w453) -> ()  [unwired: 2 in, 3 out]
                }
                frame "runWaves" {
                }
                frame "deInit" {
                }
                frame "Init" {
                }
                frame "Idle" {
                }
              }
            }
            event "Scan": Value Change {
              n101 = event-data() -> ()  [unwired: 1 in, 6 out]
            }
            event "Exposure /ms": Value Change {
              w461 = ModeEnum."generateWaves"  # Mode
              w463 = u32 2049184 items=["SENSOR MODE"=4212128, "CCD MODE"=4212384, "READOUT MODE"=4211872, "ACTIVE VIEW INDEX"=4343136, "BITS PER CHANNEL"=4342976, "IMAGE PIXEL TYPE"=4343296, "BINNING"=4215968, "EXPOSURE TIME"=2049184, "CONTRAST GAIN"=3163312, "CONTRAST OFFSET"=3163328, "LIGHT MODE"=2114720, "SENSITIVITY"=2114992, "PHOTON IMAGING MODE"=2115200, "HIGH DYNAMIC RANGE MODE"=3163360, "WHITE BALANCE"=3163568, "TEMPERATURE"=2115232, "TEMPERATURE TARGET"=2115264, "SENSOR COOLER FAN"=2115296, "LINEBUNDLE HEIGHT"=4212192, "MECHANICAL SHUTTER"=2115488, "BACK FOCUS POSITION"=8422304, "TRIGGER CONNECTOR"=1066432, "TRIGGER SOURCE"=1066144, "OUTPUT TRIGGER SOURCE"=1852576, "TRIGGER GLOBAL EXPOSURE"=2049680, "FIRST TRIGGER BEHAVIOR"=2049696, "CHANNEL SYNC"=1852352, "READOUT DIRECTION"=4211904, "PRE HSYNC COUNT"=1852704, "INTERNAL LINE SPEED"=4191408, "INTERNAL LINE INTERVAL"=4191424] ("Parameter")
              n102 = event-data() -> ()  [unwired: 1 in, 6 out]
              n103 = Bundle("Enum"=CameraControlTypeDef."Update", "Exposure /ms"="Exposure /ms", "Parameter"=w463) -> (w464:T19)  [unwired: 1 in]
              n104 = Enqueue Element(queue=w465, element=w464) -> ()  [unwired: 2 in, 3 out]
              n105 = Bundle("Mode"=w461, "Exposure /ms"="Exposure /ms") -> (w459:cluster{"Mode":T2, "Exposure /ms":dbl})  [unwired: 1 in]
              n106 = Enqueue Element(queue=w462, element=w459) -> ()  [unwired: 2 in, 3 out]
            }
          }
        }
        n107 = while {
          tunnel: w152 -> [w189]
          shift-right: [w184] -> _
          shift-left: _ -> [w183]
          tunnel: w155 -> [w182]
          tunnel: [w180] -> _
          shift-right: [w176] -> _
          shift-left: w151 -> [w175]
          shift-right: [w179] -> _
          shift-left: w154 -> [w178]
          shift-right: [w174] -> _
          shift-left: _ -> [w173]
          stop <- w188 stop-if-true
          n108 = Dequeue Element(queue=w189, timeout in ms (-1)=10) -> (queue out=w181:refnum<queue>, element=w187:T12)  [unwired: 1 in, 2 out]
          n109 = Unbundle(w187) -> ("Mode"=w186:T2, w185:T6)
          n110 = case shown="\"generateWaves\"" w186 {
            tunnel: [_ _ _ _ _ _ TRUE _ _] -> w188
            tunnel: w185 -> [_ w210 _ _ w221 _ _ _ _]
            tunnel: [w195 w200 w215 w220 w239 w257 w263 w270 w274] -> w184
            tunnel: w183 -> [w195 _ w215 w220 w239 w257 w263 w270 w274]
            tunnel: w182 -> [_ _ _ _ _ _ _ _ _]
            tunnel: w181 -> [w194 w199 w214 w219 w222 w253 w264 w269 w275]
            tunnel: [w194 w199 w214 w219 w223 w253 w264 w269 w275] -> w180
            tunnel: [w193 w196 w213 w218 w229 w256 w258 w266 w271] -> w174
            tunnel: [w190 w197 w212 w217 w231 w255 w259 w267 w272] -> w176
            tunnel: w175 -> [w191 w197 w212 w217 w225 w255 w259 w267 w272]
            tunnel: [w192 w198 w211 w216 w238 w254 w262 w268 w273] -> w179
            tunnel: w178 -> [w192 w198 w211 w216 w238 w254 w262 w268 w273]
            tunnel: w173 -> [w193 w196 w213 w218 w226 w256 w258 w266 w271]
            frame "X" {
              n111 = call "Calibration.vi"("Analogue In"=w191) -> ("Analogue In Out"=w190:refnum<k21>)
            }
            frame "XY" {
              # "XY Mirrors"
              n112 = Unbundle(w210) -> ("Piezo Position /um"=w209:dbl, "Exposure/ms"=w208:dbl, "Samples/millisecond"=w205:dbl, "Relax/ms"=w207:dbl)
              n113 = Reciprocal(x=w205) -> (1/x=w203:dbl)
              n114 = call "XY Galvo With Homography.vi"("Piezo Position (um)"=w209, "Relax (ms)"=w207, "Samples /Millisecond"=w205, "Exposure (ms)"=w208) -> ("Z Mirror Signal"=w204:dbl[], "Scan Mirror Signal"=w206:dbl[])
              n115 = Bundle By Name("Y"=w206, "dt"=w203) -> (w201:waveform(dbl))  [unwired: 1 in]
              n116 = Bundle By Name("Y"=w204, "dt"=w203) -> (w202:waveform(dbl))  [unwired: 1 in]
              n117 = Build Array(w201, w202) -> (w200:waveform(dbl)[])
            }
            frame "XYZ" {
            }
            frame "XYZT" {
            }
            frame "runWaves" {
              n118 = Unbundle By Name(w221) -> ("Samples/millisecond"=w242:dbl)  [unwired: 3 out]
              n119 = call-poly <vilib>:"DAQmx Timing.vi"("task/channels in"=w225, "rate"=w242) -> ("task out"=w241:refnum<k21>)  [unwired: 12 in, 1 out]
              n120 = call-poly <vilib>:"DAQmx Timing.vi"("task/channels in"=w226, "rate"=w242) -> ("task out"=w240:refnum<k21>)  [unwired: 12 in, 1 out]
              n121 = call-poly <vilib>:"DAQmx Write.vi"("task/channels in"=w241, "data"=w239) -> ("task out"=w237:refnum<k21>, "error out"=w234:errorcluster)  [unwired: 11 in, 1 out]
              n122 = call-poly <vilib>:"DAQmx Write.vi"("task/channels in"=w240, "data"=w238) -> ("task out"=w236:refnum<k21>, "error out"=w235:errorcluster)  [unwired: 11 in, 1 out]
              n123 = case shown="True" "Scan Continuously" {
                tunnel: w222 -> [w244 w252]
                tunnel: [w245 w251] -> w223
                tunnel: w221 -> [w246 w250]
                frame False {
                  n124 = Bundle("Mode"=ModeEnum."Idle", w246) -> (w247:T12)  [unwired: 1 in]
                  n125 = Enqueue Element(queue=w244, element=w247) -> (queue out=w245:refnum<queue>)  [unwired: 2 in, 2 out]
                }
                frame True {
                  n126 = Bundle("Mode"=ModeEnum."Idle", w250) -> (w249:T12)  [unwired: 1 in]
                  n127 = Enqueue Element(queue=w252, element=w249) -> (queue out=w251:refnum<queue>)  [unwired: 2 in, 2 out]
                }
              }
              n128 = Merge Errors(w234, w235) -> (w233:errorcluster)
              n129 = call <vilib>:"DAQmx Start Task.vi"("task/channels in"=w237, "error in"=w233) -> ("task out"=w232:refnum<k21>, "error out"=w227:errorcluster)  [unwired: 12 in]
              n130 = call <vilib>:"DAQmx Start Task.vi"("task/channels in"=w236, "error in"=w233) -> ("task out"=w230:refnum<k21>, "error out"=w228:errorcluster)  [unwired: 12 in]
              n131 = call <vilib>:"DAQmx Wait Until Done.vi"("task/channels in"=w232, "error in"=w227) -> ("task out"=w231:refnum<k21>)  [unwired: 12 in, 1 out]
              n132 = call <vilib>:"DAQmx Wait Until Done.vi"("task/channels in"=w230, "error in"=w228) -> ("task out"=w229:refnum<k21>)  [unwired: 12 in, 1 out]
            }
            frame "generateWaves" {
            }
            frame "deInit" {
              n133 = call <vilib>:"DAQmx Stop Task.vi"("task/channels in"=w259) -> ("task out"=w260:refnum<k21>, "error out"=w261:errorcluster)  [unwired: 13 in]
              n134 = call <vilib>:"DAQmx Clear Task.vi"("task in"=w260, "error in"=w261) -> ()  [unwired: 13 in, 1 out]
            }
            frame "Init" {
              # "Initialise Output Voltage Channels"
            }
            frame "Idle", Default {
            }
          }
        }
        n135 = Merge Errors(w168, w169) -> (w170:errorcluster)
      }
      frame "deinit" {
        n136 = call <vilib>:"DAQmx Stop Task.vi"("task/channels in"=w467) -> ("task out"=w468:refnum<k21>)  [unwired: 13 in, 1 out]
        n137 = call "tm_stopcapture.vi"("error in (no error)"=w479, "Handle in"=w475) -> ("error out"=w482:errorcluster, "Handle out"=w481:u32)  [unwired: 8 in]
        n138 = call <vilib>:"DAQmx Clear Task.vi"("task in"=w468) -> ()  [unwired: 14 in, 1 out]
        n139 = call "tm_unpreparecapture.vi"("error in (no error)"=w482, "Handle in"=w481) -> ("error out"=w483:errorcluster, "Handle out"=w480:u32)  [unwired: 8 in]
        n140 = call "tm_closecamera.vi"("error in (no error)"=w483, "Handle in"=w480) -> ("error out"=w484:errorcluster)  [unwired: 9 in]
        n141 = call "tm_deinitialize.vi"("error in (no error)"=w484) -> ("error out"=w485:errorcluster)  [unwired: 10 in]
        n142 = Release Queue(queue=w473, error in (no error)=w485) -> (error out=w477:errorcluster)  [unwired: 1 in, 2 out]
        n143 = Release Queue(queue=w472, error in (no error)=w485) -> (error out=w476:errorcluster)  [unwired: 1 in, 2 out]
        n144 = Merge Errors(w477, w476) -> (w478:errorcluster)
      }
    }
    n145 = Or(x="stop", y=w25) -> (x .or. y?=w26:bool)
  }
  "error IO" <- w14
  n146 = disable-structure shown="Enabled" {
    frame Disabled {
      # "Parallise decode buffer"
      n147 = call "tm_startcapture_b.vi"() -> ()  [unwired: 10 in, 2 out]
      n148 = call "tm_waitnextframe.vi"() -> ()  [unwired: 8 in, 4 out]
      n149 = call "tm_getframe_a.vi"() -> ()  [unwired: 7 in, 5 out]
    }
    frame Enabled {
    }
  }
